vi "Write Module Object.vi"(8 "error in":errorcluster, 10 "Module Information":T1 {"Module Code" format="%.0x"}, 11 "Module in":refnum<class "Module.lvclass">) -> (0 "error out":errorcluster, 3 "Module out":refnum<class "Module.lvclass">)   [LabVIEW 2015, in "SMI.lvlib" / "Module.lvclass"]
uses:
  Module.lvclass
  Controls/ModuleInformation.ctl
  Device/Device.lvclass/Device.ctl
  Device/Accessor Methods/Write Vendor Name.vi
  Device/Accessor Methods/Write Product Name.vi
  Device/Accessor Methods/Write Product ID.vi
  Device/Accessor Methods/Write Serial Number.vi
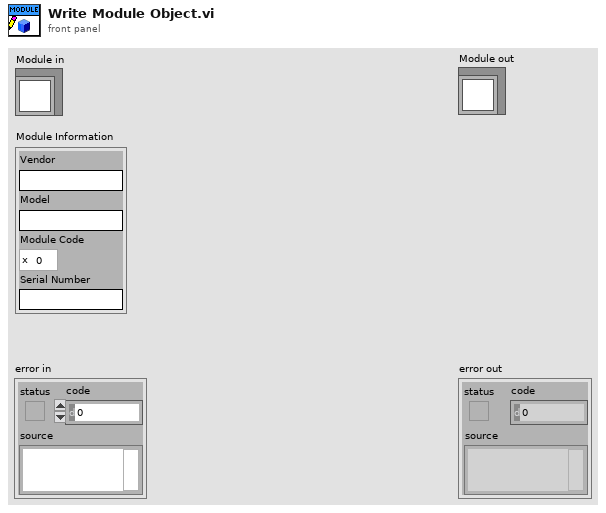
[diagram p1: front panel]
types:
  T1 = typedef "SMI.lvlib/Module.lvclass/ModuleInformation.ctl" = cluster{"Vendor":string, "Model":string, "Module Code":u16, "Serial Number":string}
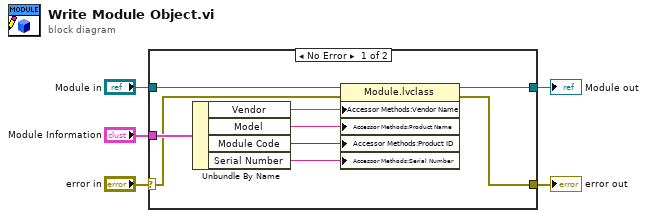
[diagram p0: block diagram]
diagram:
  n1 = case shown="No Error" "error in" {
    selector: "error in" -> [w7 w16]
    tunnel: [w6 w16] -> w4
    tunnel: [w13 w15] -> w1
    tunnel: "Module in" -> [w14 w15]
    tunnel: "Module Information" -> [w12 _]
    frame No Error {
      n2 = Unbundle By Name(w12) -> ("Vendor"=w11:string, "Model"=w10:string, "Module Code"=w9:u16, "Serial Number"=w8:string)
      n3 = property class="Module.lvclass"(reference=w14, error in=w7, "Accessor Methods:Vendor Name"=w11, "Accessor Methods:Product Name"=w10, "Accessor Methods:Product ID"=w9, "Accessor Methods:Serial Number"=w8) -> (reference out=w13:refnum<class "Module.lvclass">, error out=w6:errorcluster)
    }
    frame Error {
    }
  }
  "error out" <- w4
  "Module out" <- w1
